vi "Get Data Name_csm.vi"(8 "error in (no error)":errorcluster, 11 "Data":variant) -> (0 "error out":errorcluster, 2 "Data Name":string, 3 "Data dup":variant)   [LabVIEW 2017, in "API String Arguments Support.lvlib"]
doc: "Returns the name of the data wired on input."
uses:
  API String Arguments Support.lvlib
  <userlib>/_NEVSTOP/Communicable State Machine(CSM)/Communicable State Machine.lvlib
panel:
  # "[OpenG VI Tags] ***Do Not Remove***"
  # "Get Data Name.vi\n\nReturns the name of the data wired on input.\n\nPlease visit http://www.OpenG.org to learn about the\nOpen Source LabVIEW software movement.\n\nNOTICE -- YOU MUST LEAVE THIS NOTICE IN PLACE.  PER THE TERMS OF THE LICENSE BELOW, YOU MAY SUBLICENSE THIS SOFTWARE \nIN ANY WAY THAT DOES NOT CONFLICT WITH THIS LICENSE.\n\n### BSD License (http://www.opensource.org/licenses/bsd-license.php) Begin ###\n \nCopyright (c) 2002, Jean-Pierre Drolet <drolet_jp@hotmail.com>\nCopyright (c) 2002-2006, Jim Kring <jim@jimkring.com>\n\nAll rights reserved.\n\nRedistribution and use in source and binary forms, with or without modification, are permitted provided that the following conditions are met:\n\n    * Redistributions of source code must retain the above copyright notice, this list of conditions and the following disclaimer.\n    * Redistributions in binary form must reproduce the above copyright notice, this list of conditions and the following disclaimer in the \n       documentation and/or other materials provided with the distribution.\n    * Neither the name of SciWare, James Kring, Inc., nor the names of its contributors may be used to endorse or promote products derived \n       from this software without specific prior written permission.\n\nTHIS SOFTWARE IS PROVIDED BY THE COPYRIGHT HOLDERS AND CONTRIBUTORS \"AS IS\" AND ANY EXPRESS OR IMPLIED WARRANTIES, \nINCLUDING, BUT NOT LIMITED TO, THE IMPLIED WARRANTIES OF MERCHANTABILITY AND FITNESS FOR A PARTICULAR PURPOSE ARE \nDISCLAIMED. IN NO EVENT SHALL THE COPYRIGHT OWNER OR CONTRIBUTORS BE LIABLE FOR ANY DIRECT, INDIRECT, INCIDENTAL,\n SPECIAL, EXEMPLARY, OR CONSEQUENTIAL DAMAGES (INCLUDING, BUT NOT LIMITED TO, PROCUREMENT OF SUBSTITUTE GOODS OR \nSERVICES; LOSS OF USE, DATA, OR PROFITS; OR BUSINESS INTERRUPTION) HOWEVER CAUSED AND ON ANY THEORY OF LIABILITY, \nWHETHER IN CONTRACT, STRICT LIABILITY, OR TORT (INCLUDING NEGLIGENCE OR OTHERWISE) ARISING IN ANY WAY OUT OF THE USE \nOF THIS SOFTWARE, EVEN IF ADVISED OF THE POSSIBILITY OF SUCH DAMAGE.\n\n### BSD License End ###"
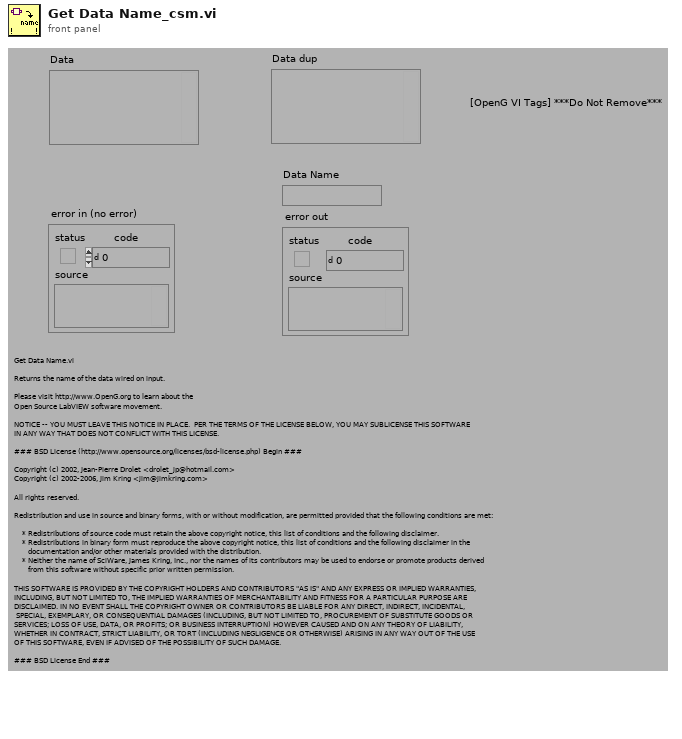
[diagram p1: front panel]
types:
  T1 = cluster{"length":u16, "private":u8, "type":enum8{"<Null>", "I8", "I16", "I32", "I64", "U8", "U16", "U32", "U64", "SGL", "DBL", "EXT", "CSG", "CDB", "CXT", "0x0F", "0x10", "0x11", "0x12", "0x13", "0x14", "Enum U8", "Enum U16", "Enum U32", "Enum U64", "SGL PQ", "DBL PQ", "EXT PQ", "CSG PQ", "CDB PQ", "CXT PQ", "0x1F", "0x20", "Boolean", "0x22", "0x23", "0x24", "0x25", "0x26", "0x27", "0x28", "0x29", "0x2A", "0x2B", "0x2C", "0x2D", "0x2E", "0x2F", "String", "0x31", "Path", "Pict", "0x34", "0x35", "0x36", "DAQ", "0x38", "0x39", "0x3A", "0x3B", "0x3C", "0x3D", "0x3E", "0x3F", "Array", "0x41", "0x42", "0x43", "0x44", "0x45", "0x46", "0x47", "0x48", "0x49", "0x4A", "0x4B", "0x4C", "0x4D", "0x4E", "0x4F", "Cluster", "0x51", "0x52", "Variant", "Waveform", "0x55", "0x56", "0x57", "0x58", "0x59", "0x5A", "0x5B", "0x5C", "0x5D", "0x5E", "Fixed Point", "0x60", "0x61", "0x62", "0x63", "0x64", "0x65", "0x66", "0x67", "0x68", "0x69", "0x6A", "0x6B", "0x6C", "0x6D", "0x6E", "0x6F", "Refnum", "0x71", "0x72", "Set Collection", "Map Collection"}, "# elements":u16}
  T2 = enum8{"<Null>", "I8", "I16", "I32", "I64", "U8", "U16", "U32", "U64", "SGL", "DBL", "EXT", "CSG", "CDB", "CXT", "0x0F", "0x10", "0x11", "0x12", "0x13", "0x14", "Enum U8", "Enum U16", "Enum U32", "Enum U64", "SGL PQ", "DBL PQ", "EXT PQ", "CSG PQ", "CDB PQ", "CXT PQ", "0x1F", "0x20", "Boolean", "0x22", "0x23", "0x24", "0x25", "0x26", "0x27", "0x28", "0x29", "0x2A", "0x2B", "0x2C", "0x2D", "0x2E", "0x2F", "String", "0x31", "Path", "Pict", "0x34", "0x35", "0x36", "DAQ", "0x38", "0x39", "0x3A", "0x3B", "0x3C", "0x3D", "0x3E", "0x3F", "Array", "0x41", "0x42", "0x43", "0x44", "0x45", "0x46", "0x47", "0x48", "0x49", "0x4A", "0x4B", "0x4C", "0x4D", "0x4E", "0x4F", "Cluster", "0x51", "0x52", "Variant", "Waveform", "0x55", "0x56", "0x57", "0x58", "0x59", "0x5A", "0x5B", "0x5C", "0x5D", "0x5E", "Fixed Point", "0x60", "0x61", "0x62", "0x63", "0x64", "0x65", "0x66", "0x67", "0x68", "0x69", "0x6A", "0x6B", "0x6C", "0x6D", "0x6E", "0x6F", "Refnum", "0x71", "0x72", "Set Collection", "Map Collection"}
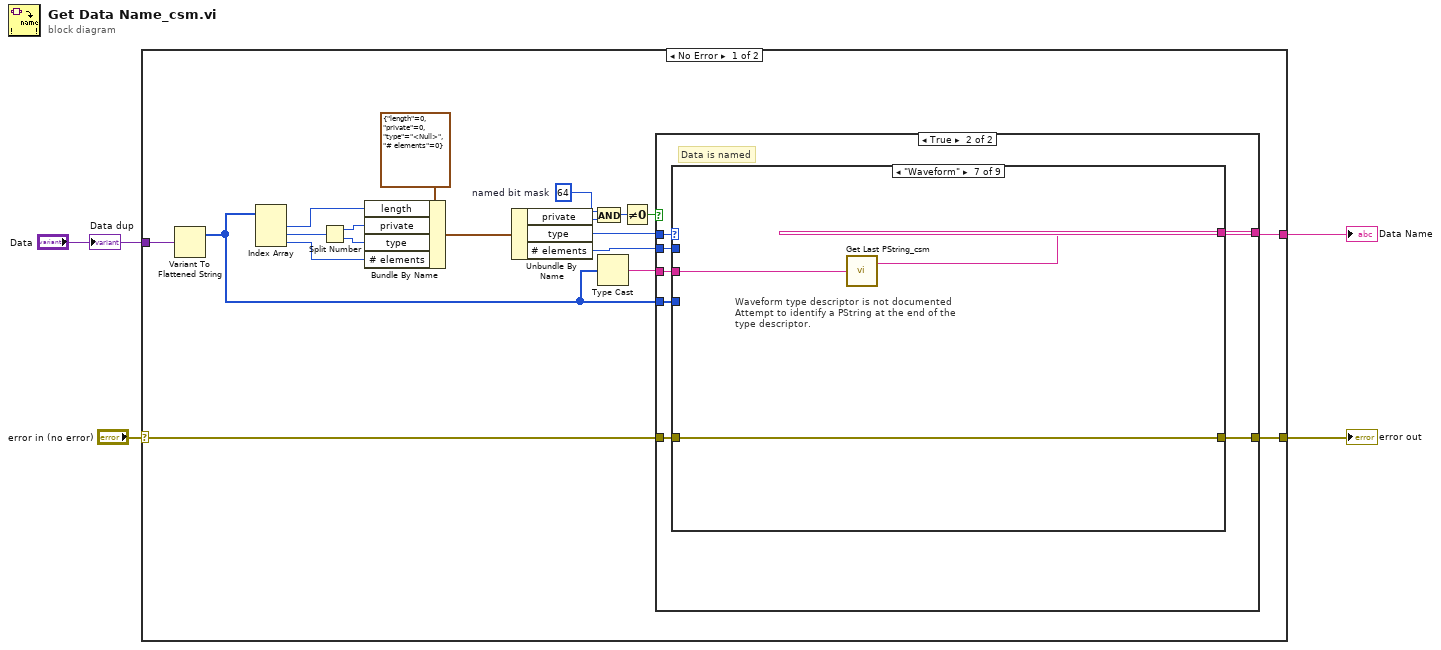
[diagram p0: block diagram]
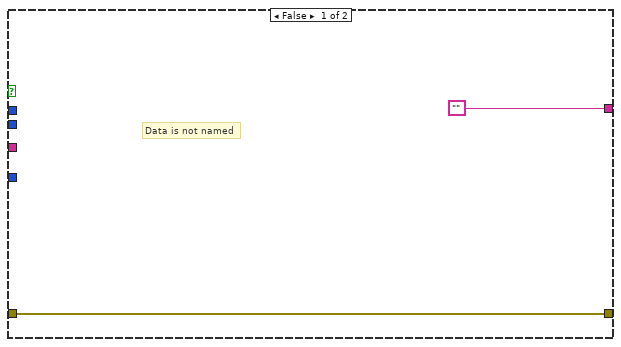
[diagram p2: hidden frame]
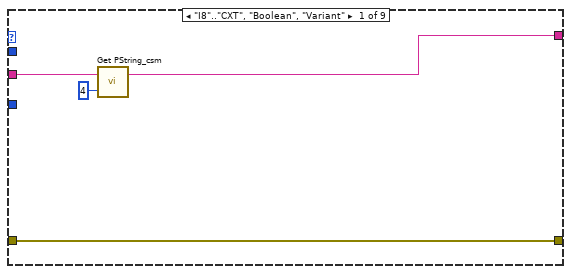
[diagram p3: hidden frame]
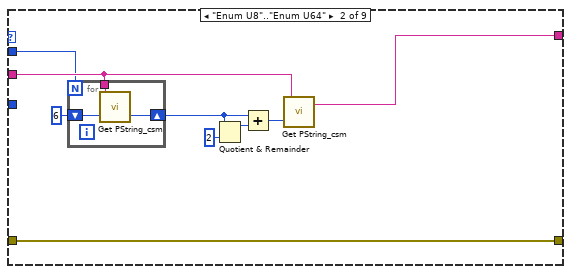
[diagram p4: hidden frame]
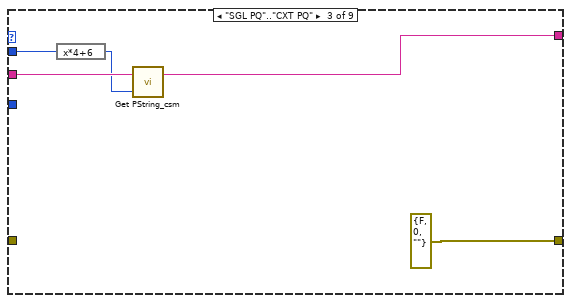
[diagram p5: hidden frame]
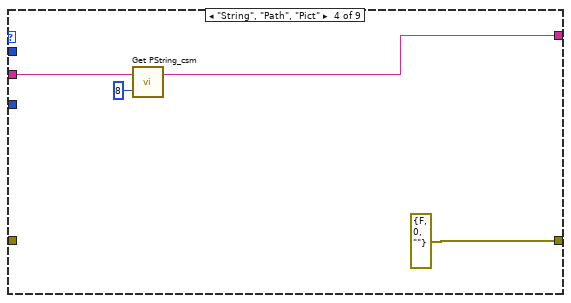
[diagram p6: hidden frame]
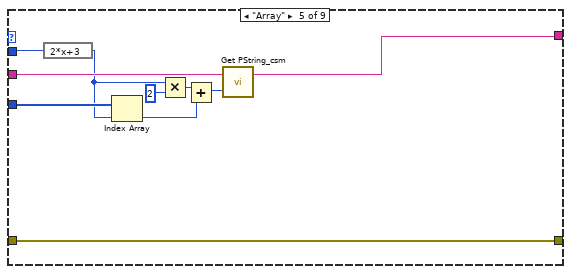
[diagram p7: hidden frame]
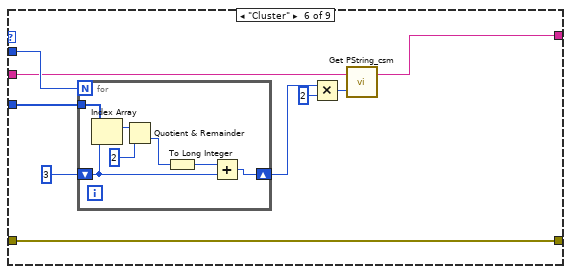
[diagram p8: hidden frame]
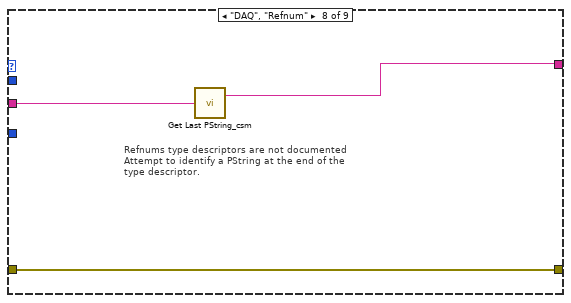
[diagram p9: hidden frame]
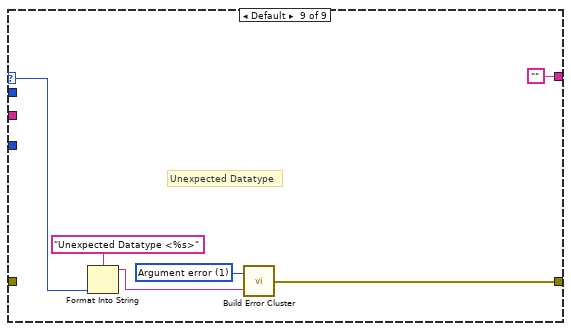
[diagram p10: hidden frame]
diagram:
  n1 = case shown="No Error" "error in (no error)" {
    selector: "error in (no error)" -> [w11 w97]
    tunnel: [w23 w97] -> w4
    tunnel: [w22 ""] -> w2
    tunnel: "Data" -> [w21 _]
    frame No Error {
      w14 = u8 64  # named bit mask
      n2 = Variant To Flattened String(Variant=w21) -> (1:w20:i16[])  [unwired: 1 out]
      n3 = Index Array(array=w20) -> (element #1=w6:i16, element #2=w9:i16, element #3=w10:i16)  [unwired: 3 in]
      n4 = Split Number(x=w9) -> (hi(x)=w7:u8, lo(x)=w8:u8)
      n5 = Bundle By Name(cluster=T1 {"length"=0, "private"=0, "type"=enum."<Null>", "# elements"=0} ("Type Descriptor Header"), "length"=w6, "private"=w7, "type"=w8, "# elements"=w10) -> (w19:T1)
      n6 = Unbundle By Name(w19) -> ("private"=w13:u8, "type"=w12:T2, "# elements"=w18:u16)
      n7 = And(x=w14, y=w13) -> (x .and. y?=w16:u8)
      n8 = Type Cast(x=w20) -> (*(type *) &x=w17:string)  [unwired: 1 in]
      n9 = Not Equal To 0?(x=w16) -> (x != 0?=w15:bool)
      n10 = case shown="True" w15 {
        tunnel: [w24 w32] -> w23
        tunnel: w12 -> [_ w31]
        tunnel: w17 -> [_ w30]
        tunnel: ["" w29] -> w22
        tunnel: w18 -> [_ w28]
        tunnel: w20 -> [_ w27]
        tunnel: w11 -> [w24 w26]
        frame False {
          # "Data is not named"
        }
        frame True {
          # "Data is named"
          n11 = case shown="\"Waveform\"" w31 {
            selector: w31 -> [_ _ _ _ _ _ _ _ w90]
            tunnel: [w33 w37 errorcluster {"status"=FALSE, "code"=0, "source"=""} ("error out") errorcluster {"status"=FALSE, "code"=0, "source"=""} ("error out") w58 w68 w84 w87 w95] -> w32
            tunnel: w30 -> [w36 w42 w52 w57 w65 w74 w86 w89 _]
            tunnel: [w34 w41 w50 w56 w64 w73 w85 w88 ""] -> w29
            tunnel: w28 -> [_ w40 w53 _ w67 w76 _ _ _]
            tunnel: w27 -> [_ _ _ _ w66 w75 _ _ _]
            tunnel: w26 -> [w33 w37 _ _ w58 w68 w84 w87 _]
            frame "I8".."CXT", "Boolean", "Variant" {
              n12 = call "Get PString_csm.vi"("offset (0)"=4, "String"=w36) -> ("PString"=w34:string)  [unwired: 1 out]
            }
            frame "Enum U8".."Enum U64" {
              n13 = for {
                N: w40 -> [_]
                tunnel: w42 -> [w46]
                shift-right: [w47] -> w44
                shift-left: 6 -> [w48]
                n14 = call "Get PString_csm.vi"("offset (0)"=w48, "String"=w46) -> ("offset past PString"=w47:i32)  [unwired: 1 out]
              }
              n15 = Quotient & Remainder(x=w44, y=2) -> (x-y*floor(x/y)=w38:i32)  [unwired: 1 out]
              n16 = Add(x=w44, y=w38) -> (x+y=w43:i32)
              n17 = call "Get PString_csm.vi"("offset (0)"=w43, "String"=w42) -> ("PString"=w41:string)  [unwired: 1 out]
            }
            frame "SGL PQ".."CXT PQ" {
              n18 = expression code="x*4+6"(w53) -> (w51:u16)
              n19 = call "Get PString_csm.vi"("offset (0)"=w51, "String"=w52) -> ("PString"=w50:string)  [unwired: 1 out]
            }
            frame "String", "Path", "Pict" {
              n20 = call "Get PString_csm.vi"("offset (0)"=8, "String"=w57) -> ("PString"=w56:string)  [unwired: 1 out]
            }
            frame "Array" {
              n21 = expression code="2*x+3"(w67) -> (w63:u16)
              n22 = Index Array(array=w66, index=w63) -> (element=w60:i16)
              n23 = Multiply(x=w63, y=u16 2) -> (x*y=w61:u16)
              n24 = Add(x=w61, y=w60) -> (x+y=w59:u16)
              n25 = call "Get PString_csm.vi"("offset (0)"=w59, "String"=w65) -> ("PString"=w64:string)  [unwired: 1 out]
            }
            frame "Cluster" {
              n26 = for {
                N: w76 -> [_]
                shift-right: [w82] -> w71
                shift-left: 3 -> [w81]
                tunnel: w75 -> [w83]
                n27 = Index Array(array=w83, index=w81) -> (element=w79:i16)
                n28 = Quotient & Remainder(x=w79, y=i16 2) -> (floor(x/y)=w80:i16)  [unwired: 1 out]
                n29 = To Long Integer(number=w80) -> (32bit integer=w77:i32)
                n30 = Add(x=w77, y=w81) -> (x+y=w82:i32)
              }
              n31 = Multiply(x=w71, y=2) -> (x*y=w70:i32)
              n32 = call "Get PString_csm.vi"("offset (0)"=w70, "String"=w74) -> ("PString"=w73:string)  [unwired: 1 out]
            }
            frame "Waveform" {
              # "Waveform type descriptor is not documented\nAttempt to identify a PString at the end of the\ntype descriptor."
              n33 = call "Get Last PString_csm.vi"("String"=w86) -> ("Last PString"=w85:string)  [unwired: 1 out]
            }
            frame "DAQ", "Refnum" {
              # "Refnums type descriptors are not documented\nAttempt to identify a PString at the end of the\ntype descriptor."
              n34 = call "Get Last PString_csm.vi"("String"=w89) -> ("Last PString"=w88:string)  [unwired: 1 out]
            }
            frame Default {
              w94 = 1 items=["No error", "Argument error", "Memory is full", "Out of zone", "End of file", "File already open", "Generic file I/O error", "File not found", "File permission error", "Disk is full", "Duplicate path", "Too many files open", "System feature not enabled", "Resource file not found", "Cannot add resource", "Resource not found", "Image not found", "Image memory error", "Pen does not exist", "Config type invalid", "Config token not found", "Config parse error", "Config memory error", "Bad external code format", "Bad external code offset", "External code not present", "Null window", "Destroy window error", "Null menu", "Print aborted", "Bad print record", "Print driver error", "Windows error during printing", "Memory error during printing", "Print dialog error", "Generic print error", "Invalid device refnum", "Device not found", "Device parameter error", "Device unit error", "Cannot open device", "Device call aborted", "Generic error", "Cancelled by user", "Object ID too low", "Object ID too high", "Object not in heap", "Unknown heap", "Unknown object (invalid DefProc)", "Unknown object (DefProc not in table)", "Message out of range", "Invalid (null) method", "Unknown message", "Manager call not supported", "Bad address", "Network operation in progress", "Network operation timed out", "Connection is busy", "Network attribute not supported", "Network error", "Address in use", "System out of memory", "Connection aborted", "Connection refused", "Not connected", "Already connected", "Connection closed", "Initialization error (interapplication manager)", "Bad occurrence", "Wait on unbound occurrence handler", "Occurrence queue overflow", "Datalog type conflict", "Unused", "Unrecognized type (interapplication manager)", "Memory corrupt", "Failed to make temporary DLL", "Old CIN version", "Drag socket not found", "Failed to load drop-object", "Failed to register OLE object", "Failed to release OLE object", "Format specifier type mismatch", "Unknown format specifier", "Too few format specifiers", "Too many format specifiers", "Scan failed", "Newer CIN version", "Error converting to variant", "Runtime menu error", "Password tampered", "Variant attribute not found", "Incompatible variant data type", "Event data is not available", "Event Store is not present", "Occurrence is not found", "Event Queue is not created", "Event info is not available", "Refnum passed is NULL", "Error retrieving Class GUID", "Error retrieving CoClass GUID", "Error retrieving TypeLib GUID.", "Bad built application magic bytes.", "Specific driver is different from the specific driver associated with the Logical Name.", "There is no session opened to the class driver.", "Max Error", "MAX - Error with config objects", "MAX - Error loading configuration", "MAX - Group not supported"]
              # "Unexpected Datatype"
              n35 = Format Into String(format string="Unexpected Datatype <%s>" ("Format String"), w90) -> (resulting string=w91:string)  [unwired: 2 in, 1 out]
              n36 = call <userlib>:"Build Error Cluster.vi"("String to Prepend to source (\"\")"=w91, "code"=w94) -> ("error out"=w95:errorcluster)
            }
          }
        }
      }
    }
    frame Error {
    }
  }
  "error out" <- w4
  "Data Name" <- w2
  "Data dup" <- "Data"
